vi "NXTwait.vi"() -> ()   [LabVIEW 2012, in "BlockParty4150.lvrbt"]
uses:
  BlockParty4150/BlockParty4150.lvrbt
  <vilib>/NXT/Subs/LVHSConnector.ctl
  <vilib>/NXT/LegoClasses/BrickReference/BrickReference.lvclass
  <vilib>/NXT/Block Support/NXT_ButtonSelector.ctl
  <vilib>/NXT/Dual Mode Library/Sensors/readNXTButton.vi
  <vilib>/NXT/Dual Mode Library/Display/drawNumber.vi
panel:
  out "NXT 2":T1
  in  "NXT":T1
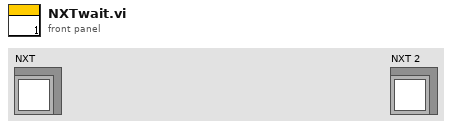
[diagram p1: front panel]
types:
  T1 = typedef "LVHSConnector.ctl" = refnum<class "BrickReference.lvclass">
  T2 = typedef "NXT_ButtonSelector.ctl" = u16
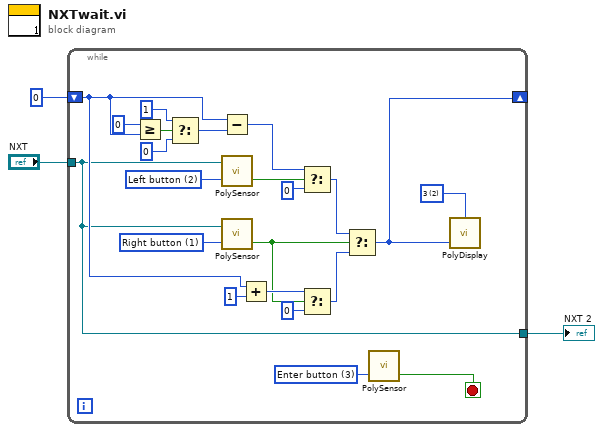
[diagram p0: block diagram]
diagram:
  n1 = while {
    tunnel: "NXT" -> [w7]
    shift-right: [w6] -> _
    shift-left: 0 -> [w8]
    tunnel: [w7] -> w1
    stop <- w24 stop-if-true
    w5 = i16 2 items=["1", "2", "3", "4", "5", "6", "7", "8"] ("Line")
    w15 = T2 1 items=["Enter button"=3, "Left button"=2, "Right button"=1] ("Button (Enter button)")
    w23 = T2 3 items=["Enter button"=3, "Left button"=2, "Right button"=1] ("Button (Enter button)")
    w25 = T2 2 items=["Enter button"=3, "Left button"=2, "Right button"=1] ("Button (Enter button)")
    n2 = Greater Or Equal?(x=0, y=w8) -> (x >= y?=w20:bool)
    n3 = Select(t=1 ("y"), s=w20, f=0) -> (s? t:f=w17:i32)
    n4 = Subtract(x=w8, y=w17) -> (x-y=w21:i32)
    n5 = call-poly <vilib>:"PolySensor.vi"("Button (Enter button)"=w25, "NXT"=w7) -> ("Yes/No"=w22:bool)  [unwired: 1 in, 1 out]
    n6 = call-poly <vilib>:"PolySensor.vi"("Button (Enter button)"=w15, "NXT"=w7) -> ("Yes/No"=w9:bool)  [unwired: 1 in, 1 out]
    n7 = Add(x=w8, y=1) -> (x+y=w14:i32)
    n8 = Select(t=w21, s=w22, f=0) -> (s? t:f=w11:i32)
    n9 = Select(t=w14, s=w9, f=0) -> (s? t:f=w10:i32)
    n10 = Select(t=w11, s=w9, f=w10) -> (s? t:f=w6:i32)
    n11 = call-poly <vilib>:"PolySensor.vi"("Button (Enter button)"=w23) -> ("Yes/No"=w24:bool)  [unwired: 2 in, 1 out]
    n12 = call-poly <vilib>:"PolyDisplay.vi"("number"=w6, "Line"=w5) -> ()  [unwired: 2 in, 1 out]
  }
  "NXT 2" <- w1
